vi "Update Tuning Matrices.vi"(8 "error in (no error)":errorcluster, 11 "Vessel in":refnum<class "Vessel.lvclass">) -> (0 "error out":errorcluster, 3 "Vessel out":refnum<class "Vessel.lvclass">)   [LabVIEW 2014, in "Vessel.lvclass"]
uses:
  Vessel.lvclass
  Controller/PID Controller/Non Linear PID Controller/Non Linear PID Controller.lvclass
  Vessel.lvclass/Vessel.ctl
  Observer/Kalman Filter/Kalman Filter.lvclass
  Supervisor/Supervisor.lvclass
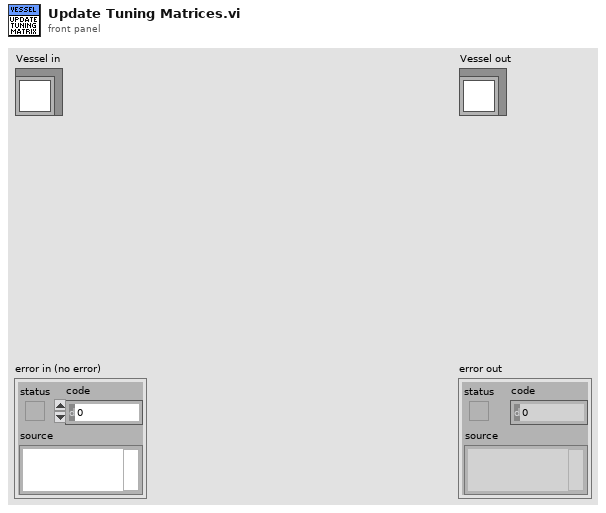
[diagram p1: front panel]
types:
  T1 = typedef "NI_Matrix.lvlib/RealMatrix.ctl" = dbl[][]
  T2 = cluster{"KP":T1, "KD":T1, "KI":T1, "KA":T1, "Update KP":bool, "Update KD":bool, "Update KI":bool, "Update KA":bool, "Name":string}
  T3 = cluster{"R":T1, "Q":T1, "Update R":bool, "Update Q":bool, "Name":string}
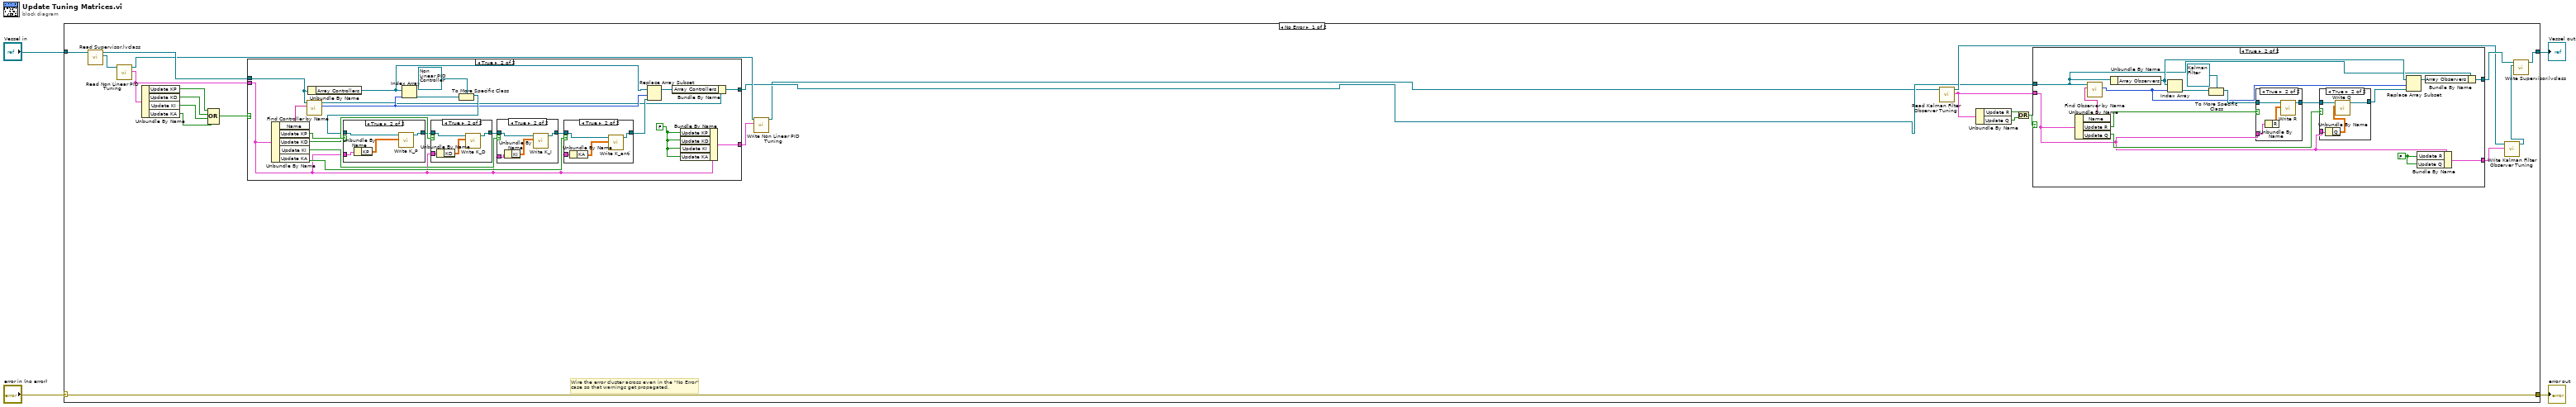
[diagram p0: block diagram]
diagram:
  n1 = case shown="No Error" "error in (no error)" {
    selector: "error in (no error)" -> [w27 w100]
    tunnel: [w27 w100] -> w3
    tunnel: [w10 w99] -> w1
    tunnel: "Vessel in" -> [w26 w99]
    frame No Error {
      # "Wire the error cluster across even in the \"No Error\"\ncase so that warnings get propagated."
      n2 = call "Read Supervisor.lvclass.vi"("Vessel in"=w26) -> ("Supervisor.lvclass"=w25:refnum<class "Supervisor.lvclass">, "Vessel out"=w14:refnum<class "Vessel.lvclass">)  [unwired: 8 in, 1 out]
      n3 = call-dynamic "Read Non Linear PID Tuning.vi"("Supervisor in"=w25) -> ("Non Linear PID Tuning"=w24:T2, "Supervisor out"=w12:refnum<class "Supervisor.lvclass">)  [unwired: 8 in, 1 out]
      n4 = Unbundle By Name(w24) -> ("Update KP"=w23:bool, "Update KD"=w22:bool, "Update KI"=w21:bool, "Update KA"=w20:bool)
      n5 = Compound Arithmetic op=OR(w23, w22, w21, w20) -> (w19:bool)
      n6 = case shown="True" w19 {
        tunnel: w24 -> [w56 w61]
        tunnel: w14 -> [w57 w78]
        tunnel: [w57 w62] -> w6
        tunnel: [w56 w59] -> w13
        frame False {
        }
        frame True {
          w60 = FALSE
          n7 = Unbundle By Name(w61) -> ("Name"=w58:string, "Update KP"=w77:bool, "Update KD"=w76:bool, "Update KI"=w75:bool, "Update KA"=w74:bool)
          n8 = call-dynamic "Find Controller by Name.vi"("Controller Name"=w58, "Vessel in"=w78) -> ("Index"=w67:i32, "Vessel out"=w64:refnum<class "Vessel.lvclass">)  [unwired: 7 in, 1 out]
          n9 = Unbundle By Name(w78) -> ("Array Controllers"=w66:refnum<class "Controller.lvclass">[])
          n10 = Index Array(array=w66, index=w67) -> (element=w73:refnum<class "Controller.lvclass">)
          n11 = To More Specific Class(target class=refnum<class "Non Linear PID Controller.lvclass"> refnum ("Controller Library:Non Linear PID Controller.lvclass"), reference=w73) -> (specific class reference=w71:refnum<class "Non Linear PID Controller.lvclass">)  [unwired: 1 in, 1 out]
          n12 = case shown="True" w77 {
            tunnel: w71 -> [w94 w96]
            tunnel: [w94 w95] -> w70
            tunnel: w61 -> [_ w98]
            frame False {
            }
            frame True {
              n13 = Unbundle By Name(w98) -> ("KP"=w97:T1)
              n14 = call-dynamic "Write K_P.vi"("Real Matrix"=w97, "PID Controller in"=w96) -> ("PID Controller out"=w95:refnum<class "Non Linear PID Controller.lvclass">)  [unwired: 8 in, 1 out]
            }
          }
          n15 = case shown="True" w76 {
            tunnel: w70 -> [w89 w91]
            tunnel: [w89 w90] -> w69
            tunnel: w61 -> [_ w93]
            frame False {
            }
            frame True {
              n16 = Unbundle By Name(w93) -> ("KD"=w92:T1)
              n17 = call-dynamic "Write K_D.vi"("Real Matrix"=w92, "PID Controller in"=w91) -> ("PID Controller out"=w90:refnum<class "Non Linear PID Controller.lvclass">)  [unwired: 8 in, 1 out]
            }
          }
          n18 = case shown="True" w75 {
            tunnel: w69 -> [w84 w86]
            tunnel: [w84 w85] -> w68
            tunnel: w61 -> [_ w88]
            frame False {
            }
            frame True {
              n19 = Unbundle By Name(w88) -> ("KI"=w87:T1)
              n20 = call-dynamic "Write K_I.vi"("Real Matrix"=w87, "PID Controller in"=w86) -> ("PID Controller out"=w85:refnum<class "Non Linear PID Controller.lvclass">)  [unwired: 8 in, 1 out]
            }
          }
          n21 = case shown="True" w74 {
            tunnel: w68 -> [w79 w81]
            tunnel: [w79 w80] -> w65
            tunnel: w61 -> [_ w83]
            frame False {
            }
            frame True {
              n22 = Unbundle By Name(w83) -> ("KA"=w82:T1)
              n23 = call-dynamic "Write K_anti.vi"("Real Matrix"=w82, "Non Linear PID Controller in"=w81) -> ("Non Linear PID Controller out"=w80:refnum<class "Non Linear PID Controller.lvclass">)  [unwired: 8 in, 1 out]
            }
          }
          n24 = Replace Array Subset(array=w66, new element=w65, index=w67) -> (w63:refnum<class "Controller.lvclass">[])
          n25 = Bundle By Name(cluster=w64, "Array Controllers"=w63) -> (w62:refnum<class "Vessel.lvclass">)
          n26 = Bundle By Name(cluster=w61, "Update KP"=w60, "Update KD"=w60, "Update KI"=w60, "Update KA"=w60) -> (w59:T2)
        }
      }
      n27 = call-dynamic "Write Non Linear PID Tuning.vi"("Non Linear PID Tuning"=w13, "Supervisor in"=w12) -> ("Supervisor out"=w5:refnum<class "Supervisor.lvclass">)  [unwired: 8 in, 1 out]
      n28 = call-dynamic "Read Kalman Filter Observer Tuning.vi"("Supervisor in"=w5) -> ("Kalman Filter Observer Tuning"=w15:T3, "Supervisor out"=w7:refnum<class "Supervisor.lvclass">)  [unwired: 8 in, 1 out]
      n29 = Unbundle By Name(w15) -> ("Update R"=w18:bool, "Update Q"=w17:bool)
      n30 = Or(x=w18, y=w17) -> (x .or. y?=w16:bool)
      n31 = case shown="True" w16 {
        tunnel: w15 -> [w28 w33]
        tunnel: w6 -> [w29 w36]
        tunnel: [w29 w34] -> w9
        tunnel: [w28 w31] -> w11
        frame False {
        }
        frame True {
          w32 = FALSE
          n32 = Unbundle By Name(w33) -> ("Name"=w30:string, "Update R"=w43:bool, "Update Q"=w42:bool)
          n33 = call-dynamic "Find Observer by Name.vi"("Observer Name"=w30, "Vessel in"=w36) -> ("Index"=w37:i32)  [unwired: 7 in, 2 out]
          n34 = Unbundle By Name(w36) -> ("Array Observers"=w39:refnum<class "Observer.lvclass">[])
          n35 = Index Array(array=w39, index=w37) -> (element=w45:refnum<class "Observer.lvclass">)
          n36 = To More Specific Class(target class=refnum<class "Kalman Filter.lvclass"> refnum ("Observer Library.lvlib:Kalman Filter.lvclass"), reference=w45) -> (specific class reference=w41:refnum<class "Kalman Filter.lvclass">)  [unwired: 1 in, 1 out]
          n37 = case shown="True" w43 {
            tunnel: w33 -> [_ w53]
            tunnel: w41 -> [w51 w55]
            tunnel: [w51 w54] -> w40
            frame False {
            }
            frame True {
              n38 = Unbundle By Name(w53) -> ("R"=w52:T1)
              n39 = call-dynamic "Write R.vi"("Real Matrix"=w52, "Kalman Filter in"=w55) -> ("Kalman Filter out"=w54:refnum<class "Kalman Filter.lvclass">)  [unwired: 8 in, 1 out]
            }
          }
          n40 = case shown="True" w42 {
            tunnel: w33 -> [_ w48]
            tunnel: w40 -> [w46 w50]
            tunnel: [w46 w49] -> w38
            frame False {
            }
            frame True {
              n41 = Unbundle By Name(w48) -> ("Q"=w47:T1)
              n42 = call-dynamic "Write Q.vi"("Real Matrix"=w47, "Kalman Filter in"=w50) -> ("Kalman Filter out"=w49:refnum<class "Kalman Filter.lvclass">)  [unwired: 8 in, 1 out]
            }
          }
          n43 = Replace Array Subset(array=w39, new element=w38, index=w37) -> (w35:refnum<class "Observer.lvclass">[])
          n44 = Bundle By Name(cluster=w33, "Update R"=w32, "Update Q"=w32) -> (w31:T3)
          n45 = Bundle By Name(cluster=w36, "Array Observers"=w35) -> (w34:refnum<class "Vessel.lvclass">)
        }
      }
      n46 = call-dynamic "Write Kalman Filter Observer Tuning.vi"("Kalman Filter Observer Tuning"=w11, "Supervisor in"=w7) -> ("Supervisor out"=w8:refnum<class "Supervisor.lvclass">)  [unwired: 8 in, 1 out]
      n47 = call "Write Supervisor.lvclass.vi"("Supervisor.lvclass"=w8, "Vessel in"=w9) -> ("Vessel out"=w10:refnum<class "Vessel.lvclass">)  [unwired: 8 in, 1 out]
    }
    frame Error {
    }
  }
  "error out" <- w3
  "Vessel out" <- w1
